vi "click_mouse_at_location.vi"(8 "error in":errorcluster, 11 "position":cluster{"x posns":i32, "y posns":i32}) -> (0 "error out":errorcluster, 3 "position":cluster{i32, i32})   [LabVIEW 2018]
uses:
  User32.dll
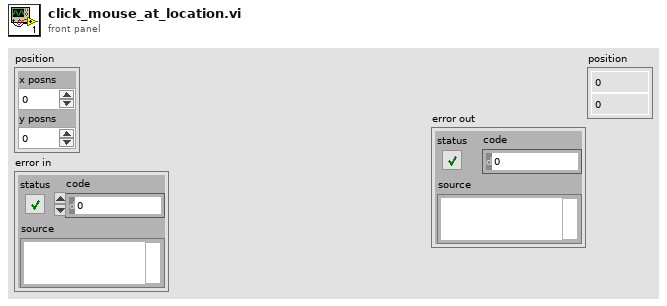
[diagram p1: front panel]
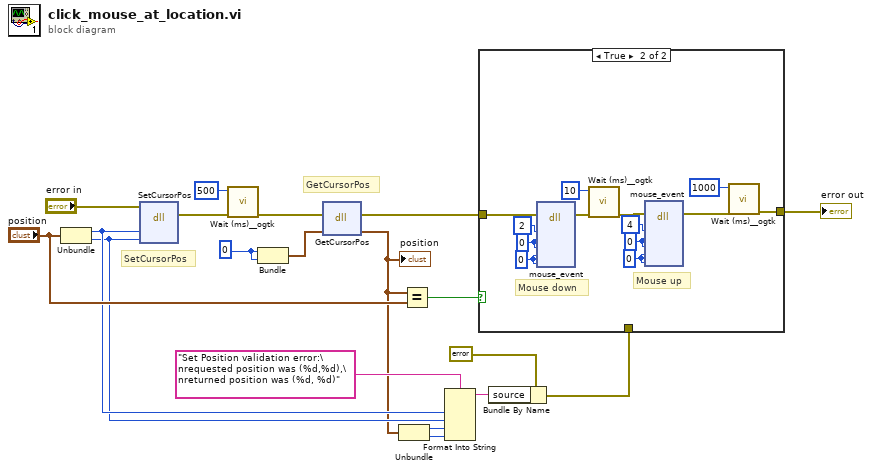
[diagram p0: block diagram]
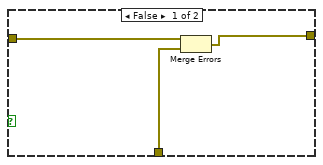
[diagram p2: hidden frame]
diagram:
  w18 = 0
  # "GetCursorPos"
  # "SetCursorPos"
  n1 = Unbundle("position") -> ("x posns"=w8:i32, "y posns"=w7:i32)
  n2 = dll-call lib="User32.dll" fn="SetCursorPos"(error in="error in", w8, w7) -> (error out=w16:errorcluster)  [unwired: 5 in, 1 out]
  n3 = call <userlib>:"Wait (ms)__ogtk.vi"("error in (no error)"=w16, "milliseconds to wait"=u32 500) -> ("error out"=w14:errorcluster)  [unwired: 8 in, 1 out]
  n4 = Bundle(w18, w18) -> (w17:cluster{i32, i32})  [unwired: 1 in]
  n5 = dll-call lib="User32.dll" fn="GetCursorPos"(error in=w14, "position"=w17) -> (error out=w13:errorcluster, "position"=w6:cluster{i32, i32})  [unwired: 3 in, 1 out]
  "position" <- w6
  n6 = Unbundle(w6) -> (w5:i32, w4:i32)
  n7 = Equal?(x=w6, y="position") -> (x = y?=w11:bool)
  n8 = Format Into String(format string="Set Position validation error:\nrequested position was (%d,%d),\nreturned position was (%d, %d)" ("source"), w8, w7, w5, w4) -> (resulting string=w9:string)  [unwired: 2 in, 1 out]
  n9 = Bundle By Name(cluster=errorcluster {"status"=TRUE, "code"=0, "source"=""} ("error out"), "source"=w9) -> (w2:errorcluster)
  n10 = case shown="True" w11 {
    tunnel: [w20 w35] -> w19
    tunnel: w13 -> [w22 w23]
    tunnel: w2 -> [w21 _]
    frame False {
      n11 = Merge Errors(w22, w21) -> (w20:errorcluster)
    }
    frame True {
      w29 = 0 ("dwExtraInfo")
      w30 = u32 0 ("dwExtraInfo")
      w32 = 0 ("dwExtraInfo")
      w33 = u32 0 ("dwExtraInfo")
      # "Mouse up"
      # "Mouse down"
      n12 = dll-call lib="user32.dll" fn="mouse_event" ("Mouse_Event")(error in=w23, "dwFlags"=2, "dx"=w32, "dy"=w32, "dwData"=w33, "dwExtraInfo"=w33) -> (error out=w27:errorcluster)  [unwired: 8 in, 1 out]
      n13 = call <userlib>:"Wait (ms)__ogtk.vi"("error in (no error)"=w27, "milliseconds to wait"=u32 10) -> ("error out"=w26:errorcluster)  [unwired: 8 in, 1 out]
      n14 = dll-call lib="user32.dll" fn="mouse_event" ("Mouse_Event")(error in=w26, "dwFlags"=4, "dx"=w29, "dy"=w29, "dwData"=w30, "dwExtraInfo"=w30) -> (error out=w24:errorcluster)  [unwired: 8 in, 1 out]
      n15 = call <userlib>:"Wait (ms)__ogtk.vi"("error in (no error)"=w24, "milliseconds to wait"=u32 1000) -> ("error out"=w35:errorcluster)  [unwired: 8 in, 1 out]
    }
  }
  "error out" <- w19
